vi "Get Name Priv.vi"(8 "error in":errorcluster, 10 "Unique ID":string, 11 "Tree Dictionary":variant) -> (0 "error out":errorcluster, 1 "Name":string, 3 "Tree Dictionary Out":variant)   [LabVIEW 2020, in "NI_VIAnCFGDataStructure.lvlib" / "Tree.lvclass"]
uses:
  <vilib>/addons/analyzer/VIAnCFGDataStructure/Tree Manager/Tree.lvclass
  <vilib>/addons/analyzer/VIAnCFGDataStructure/Tree Manager/Typedefs/Tree Cluster.ctl
  <vilib>/Utility/error.llb/Error Cluster From Error Code.vi
  <vilib>/ErrorRing/Error Ring.xnode
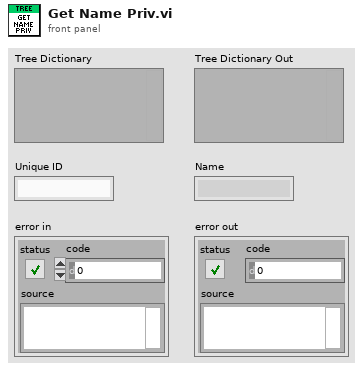
[diagram p1: front panel]
types:
  T1 = typedef "NI_VIAnCFGDataStructure.lvlib/Tree.lvclass/Tree Cluster.ctl" = cluster{"Unique ID":string, "Parent ID":string, "Child IDs":string[], "Name":string, "MetaData":string, "Data IDs":string[]}
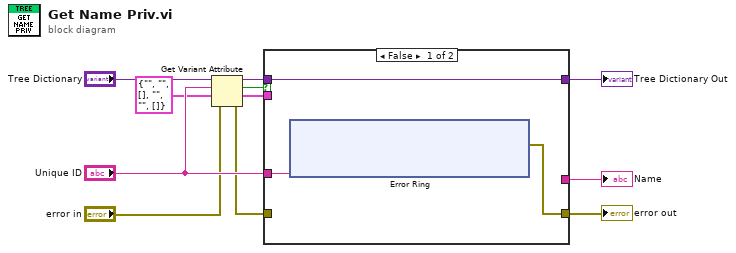
[diagram p0: block diagram]
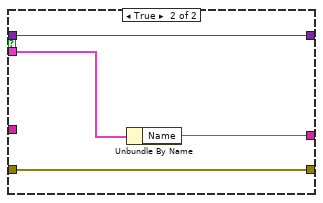
[diagram p2: hidden frame]
diagram:
  n1 = Get Variant Attribute(Variant="Tree Dictionary", name="Unique ID", default value (empty Variant)=T1 {"Unique ID"="", "Parent ID"="", "Child IDs"=[], "Name"="", "MetaData"="", "Data IDs"=[]} ("Cluster of class private data"), error in="error in") -> (duplicate Variant=w2:variant, found=w4:bool, value=w3:T1, error out=w1:errorcluster)
  n2 = case shown="False" w4 {
    tunnel: w3 -> [_ w23]
    tunnel: w2 -> [w14 w25]
    tunnel: w1 -> [_ w24]
    tunnel: [w13 w24] -> w9
    tunnel: [w14 w25] -> w7
    tunnel: "Unique ID" -> [w12 _]
    tunnel: [_ w22] -> w11
    frame False {
      n3 = xnode "Error Ring"("parameter 0"=w12) -> ("error out"=w13:errorcluster)
    }
    frame True {
      n4 = Unbundle By Name(w23) -> ("Name"=w22:string)
    }
  }
  "Name" <- w11
  "error out" <- w9
  "Tree Dictionary Out" <- w7
